vi "GETRequest.vi"(8 "error in (no error)":errorcluster, 9 "Parameter":string, 10 "Request":string, 11 "ByteGSAPIBase":refnum<class "ByteGSAPIBase.lvclass">) -> (0 "error out":errorcluster, 1 "Headers":string, 2 "Body":string, 3 "ByteGSAPIBase 2":refnum<class "ByteGSAPIBase.lvclass">)   [LabVIEW 2019, in "ByteGSWebAPI.lvlib" / "ByteGSAPIBase.lvclass"]
doc: "Effettua una richiesta di GET al server come:\nSERVER/api/bytegs/RICHIESTA/PARAMETRO(opzionale)"
uses:
  ByteGSAPIBase.lvclass
  Status_Code.ctl
  ByteGSAPIBase.lvclass/ByteGSAPIBase.ctl
  <vilib>/httpClient/LabVIEWHTTPClient.lvlib
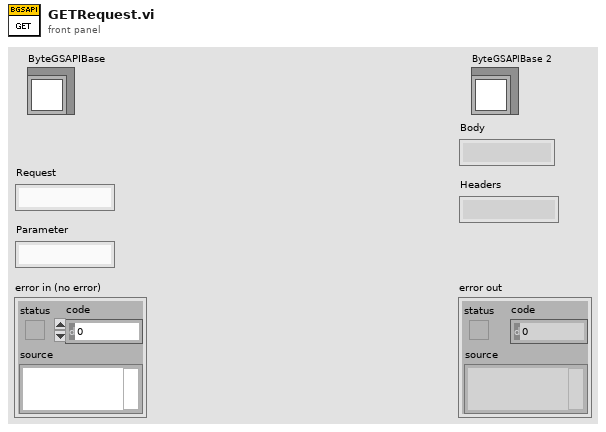
[diagram p1: front panel]
types:
  T1 = typedef "ByteGSWebAPI.lvlib/ByteGSAPIBase.lvclass/Status_Code.ctl" = u16
  T2 = typedef "LabVIEWHTTPClient.lvlib/ClientHandle.ctl" = refnum<k1>
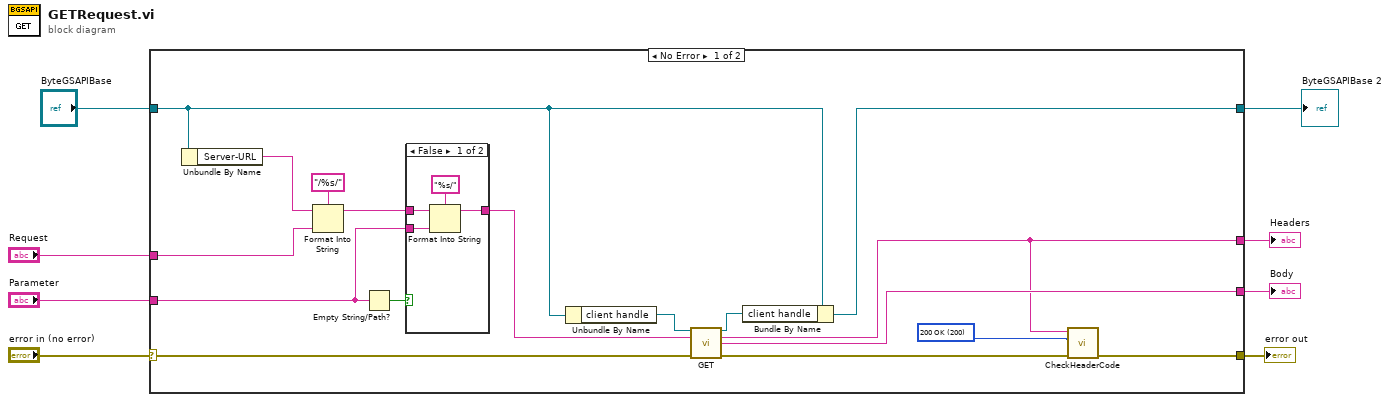
[diagram p0: block diagram]
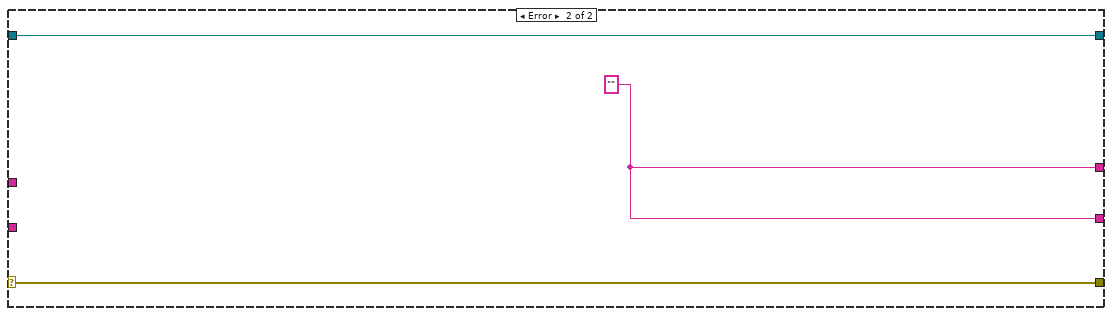
[diagram p3: hidden frame]
diagram:
  n1 = case shown="No Error" "error in (no error)" {
    selector: "error in (no error)" -> [w21 w33]
    tunnel: [w9 w33] -> w7
    tunnel: [w18 w32] -> w1
    tunnel: "ByteGSAPIBase" -> [w15 w32]
    tunnel: "Request" -> [w13 _]
    tunnel: "Parameter" -> [w22 _]
    tunnel: [w17 w31] -> w4
    tunnel: [w10 w31] -> w3
    frame No Error {
      w11 = T1 200 items=["200 OK"=200, "201 Created"=201, "400 Bad Request"=400, "401 Unauthorized"=401, "403 Forbidden"=403, "404 Not Found"=404, "405 Method Not Allowed"=405, "406 Not Acceptable"=406, "500 Internal Server Error"=500] ("Code")
      n2 = Unbundle By Name(w15) -> ("Server-URL"=w14:string)
      n3 = Format Into String(format string="/%s/" ("url"), initial string=w14, w13) -> (resulting string=w24:string)  [unwired: 1 in, 1 out]
      n4 = Empty String/Path?(string/path=w22) -> (empty?=w23:bool)
      n5 = case shown="False" w23 {
        tunnel: w24 -> [w28 w30]
        tunnel: [w26 w30] -> w20
        tunnel: w22 -> [w27 _]
        frame False {
          n6 = Format Into String(format string="%s/" ("url"), initial string=w28, w27) -> (resulting string=w26:string)  [unwired: 1 in, 1 out]
        }
        frame True {
        }
      }
      n7 = Unbundle By Name(w15) -> ("client handle"=w19:T2)
      n8 = call <vilib>:"GET.vi"("client handle"=w19, "url"=w20, "error in (no error)"=w21) -> ("client handle out"=w16:T2, "headers"=w10:string, "body"=w17:string, "error out"=w12:errorcluster)  [unwired: 9 in]
      n9 = Bundle By Name(cluster=w15, "client handle"=w16) -> (w18:refnum<class "ByteGSAPIBase.lvclass">)
      n10 = call "CheckHeaderCode.vi"("error in (no error)"=w12, "Expected code (200)"=w11, "Headers"=w10) -> ("error out"=w9:errorcluster)  [unwired: 8 in]
    }
    frame Error {
      w31 = "" ("body")
    }
  }
  "error out" <- w7
  "Body" <- w4
  "Headers" <- w3
  "ByteGSAPIBase 2" <- w1
